vi "MessungKlimadaten(SubVI).vi"(7 "Boolesch":bool, 8 "Fehler (Eingang, kein Fehler)":errorcluster, 9 "VISA resource name out":refnum<visa-resource-name>, 10 "Lufttemperatur [°C] (Eingang)":refnum<vi>, 11 "Luftdruck [mbar] (Eingang)":refnum<vi>) -> (0 "Fehler (Ausgang)":errorcluster, 3 "VISA-Referenz (Ausgang)":refnum<visa-resource-name>)   [LabVIEW 2014]
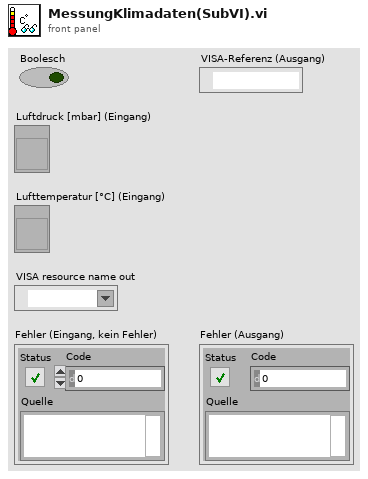
[diagram p1: front panel]
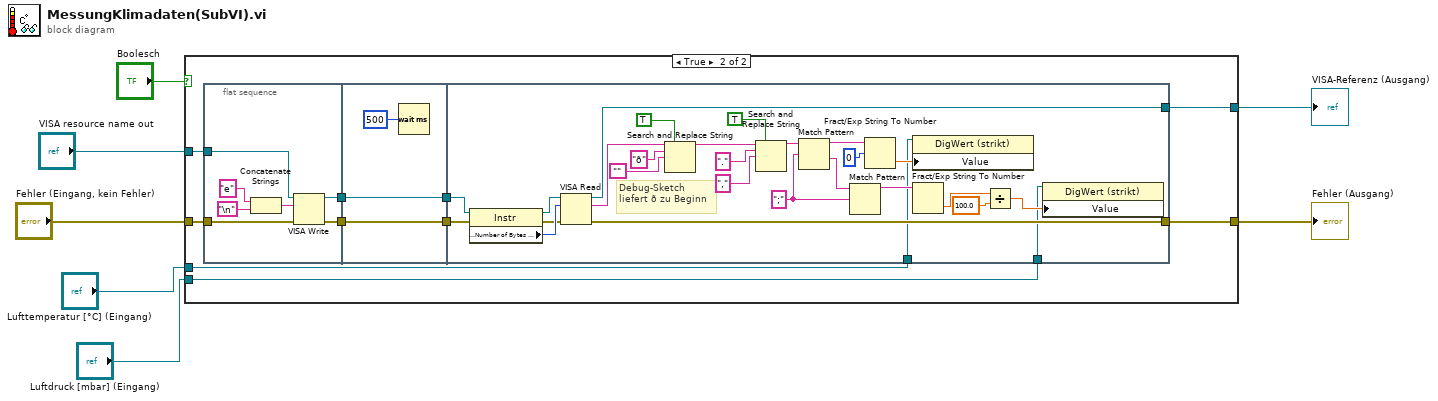
[diagram p0: block diagram]
diagram:
  n1 = case shown="True" "Boolesch" {
    tunnel: [w9 w12] -> w3
    tunnel: [w8 w13] -> w4
    tunnel: "VISA resource name out" -> [w9 w19]
    tunnel: "Fehler (Eingang, kein Fehler)" -> [w8 w18]
    tunnel: "Luftdruck [mbar] (Eingang)" -> [_ w11]
    tunnel: "Lufttemperatur [°C] (Eingang)" -> [_ w10]
    frame False {
    }
    frame True {
      n2 = flat-sequence {
        tunnel: w19 -> [w24]
        tunnel: w18 -> [w23]
        tunnel: [w26] -> w17
        tunnel: [w25] -> w16
        tunnel: w17 -> [w29]
        tunnel: w16 -> [w28]
        tunnel: [w29] -> w15
        tunnel: [w28] -> w14
        tunnel: w15 -> [w41]
        tunnel: w14 -> [w40]
        tunnel: [w43] -> w13
        tunnel: [w42] -> w12
        tunnel: w11 -> [w39]
        tunnel: w10 -> [w38]
        frame #0 {
          n3 = Concatenate Strings("e" ("String"), "\n") -> (w22:string)
          n4 = VISA Write(VISA resource name=w24, write buffer=w22, error in (no error)=w23) -> (VISA resource name out=w26:refnum<visa-resource-name>, error out=w25:errorcluster)  [unwired: 1 out]
        }
        frame #1 {
          n5 = Wait (ms)(milliseconds to wait=u32 500 ("Zu wartende ms")) -> ()  [unwired: 1 out]
        }
        frame #2 {
          w47 = ";" ("Regulärer Ausdruck")
          # "Debug-Sketch liefert ð zu Beginn"
          n6 = property class="Instr"(reference=w41, error in=w40) -> (reference out=w48:refnum<visa-resource-name>, error out=w49:errorcluster, "Serial Settings:Number of Bytes at Serial Port"=w50:u32)
          n7 = VISA Read(VISA resource name=w48, byte count=w50, error in (no error)=w49) -> (VISA resource name out=w42:refnum<visa-resource-name>, read buffer=w30:string, error out=w43:errorcluster)  [unwired: 1 out]
          n8 = Search and Replace String(replace all?=TRUE ("Alle ersetzen? (F)"), input string=w30, search string="ð" ("Such-String"), replace string="") -> (result string=w32:string)  [unwired: 4 in, 3 out]
          n9 = Search and Replace String(replace all?=TRUE ("Alle ersetzen? (F)"), input string=w32, search string="." ("Such-String"), replace string="," ("Ersetzungs-String (\"\")")) -> (result string=w54:string)  [unwired: 4 in, 3 out]
          n10 = Match Pattern(string=w54, regular expression=w47) -> (before substring=w35:string, after substring=w55:string)  [unwired: 1 in, 2 out]
          n11 = Match Pattern(string=w55, regular expression=w47) -> (before substring=w56:string)  [unwired: 1 in, 3 out]
          n12 = Fract/Exp String To Number(string=w35, offset=0 ("Offset")) -> (number=w51:dbl)  [unwired: 2 in, 1 out]
          n13 = property class="DigWert (strikt)"(reference=w38, "Value"=w51) -> ()  [unwired: 1 in, 2 out]
          n14 = Fract/Exp String To Number(string=w56) -> (number=w53:dbl)  [unwired: 3 in, 1 out]
          n15 = Divide(x=w53, y=100.0 ("x")) -> (x/y=w52:dbl)
          n16 = property class="DigWert (strikt)"(reference=w39, "Value"=w52) -> ()  [unwired: 1 in, 2 out]
        }
      }
    }
  }
  "Fehler (Ausgang)" <- w4
  "VISA-Referenz (Ausgang)" <- w3
